vi "Reset Quadrature.vi"(6 "error in":errorcluster, 8 "Reverse?":bool=TRUE, 9 "Forward Position":i32, 10 "Module Number":enum16{"1", "2", "3", "4"}(ring), 11 "CAN Talon SRX Ref":T1={"DeviceStatus"={"status"=FALSE, "code"=0, "source"=""}, "Type"=enum."PWM", "PWM"={"PWM Channel"=enum."PWM 1", "DeadBand"={"Name"="", "maxPositivePwm"=0, "minPositivePwm"=0, "centerPwm"=0, "maxNegativePwm"=0, "minNegativePwm"=0, "angularRange"=0}}, "CAN"={"Device Number"=0, "SetOutput VI Ref"=variant(enum8{"Percent VBus", "Current", "Speed", "Position", "Voltage"} enum."Percent VBus"), "GetOutput VI Ref"=variant(refnum<k1> refnum), "Enable VI Ref"=variant(dbl 12.0), "Disable VI Ref"=variant(enum8{"Percent VBus", "Speed", "Position", "Slave", "Unchanged / Invalid", "Voltage Compensation", "Current", "Motion Profile"} enum."Percent VBus"), "Data"=variant}, "Invert"=FALSE, "DIO PWM"={"PWM \"Enable\" Channel"=enum."Invalid", "DIOChannel"=enum."Invalid", "PWM Rate"=0.0}}) -> (0 "error out":errorcluster, 2 "Motor Output":dbl)   [LabVIEW 2017, in "Huskie Swerve.lvlib"]
uses:
  Huskie Swerve.lvlib
  <vilib>/Rock Robotics/WPI/MotorControl/WPI_MotorControlDeviceRef.ctl
  <vilib>/Rock Robotics/WPI/MotorControl/WPI_MotorControlType.ctl
  <vilib>/Rock Robotics/SystemInterfaces/DIO/FPGA_DIOPWMChannel.ctl
  <vilib>/Rock Robotics/WPI/PWM/WPI_PWMDeadband.ctl
  <vilib>/Rock Robotics/SystemInterfaces/DIO/FPGA_DIOChannel.ctl
  <vilib>/Rock Robotics/WPI/ThirdParty/Phoenix-LabVIEW/Motor Controller/Controls/CTRE_Phoenix_MotorControl_ControlMode.ctl
  <vilib>/Rock Robotics/WPI/ThirdParty/Phoenix-LabVIEW/Motor Controller/Get/CTRE_Phoenix_MotorController_GetPulseWidthAll.vi
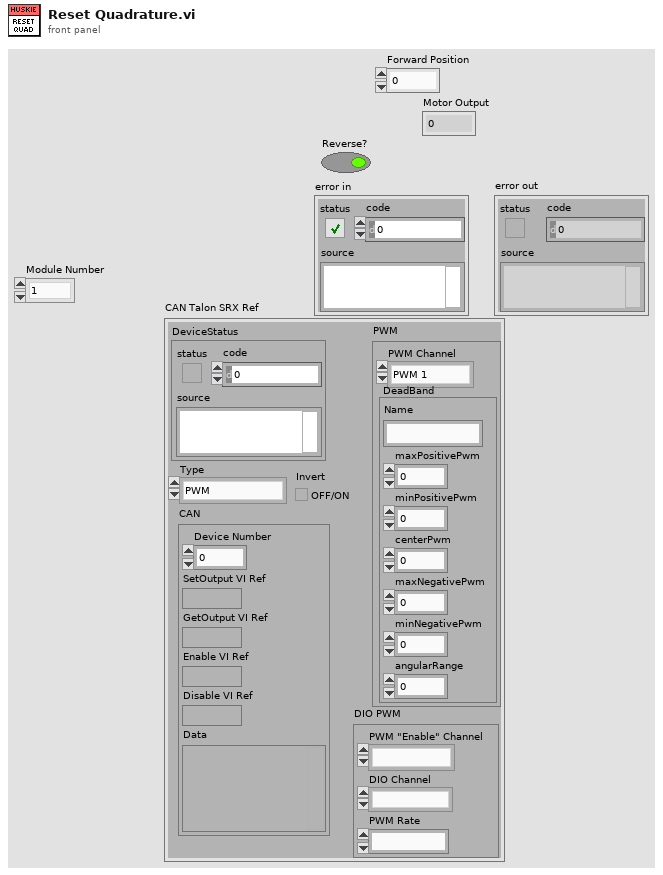
[diagram p1: front panel]
types:
  T1 = typedef "WPI_MotorControlDeviceRef.ctl" = cluster{"DeviceStatus":errorcluster, "Type":T2, "PWM":cluster{"PWM Channel":T3, "DeadBand":T4}, "CAN":cluster{"Device Number":u8, "SetOutput VI Ref":variant, "GetOutput VI Ref":variant, "Enable VI Ref":variant, "Disable VI Ref":variant, "Data":variant}, "Invert":bool, "DIO PWM":cluster{"PWM \"Enable\" Channel":T3, "DIOChannel":T5, "PWM Rate":dbl}}
  T2 = typedef "WPI_MotorControlType.ctl" = enum16{"PWM", "CAN", "DIO PWM"}
  T3 = typedef "FPGA_DIOPWMChannel.ctl" = enum8{"PWM 0", "PWM 1", "PWM 2", "PWM 3", "PWM 4", "PWM 5", "PWM 6", "PWM 7", "PWM 8", "PWM 9", "PWM MXP 0", "PWM MXP 1", "PWM MXP 2", "PWM MXP 3", "PWM MXP 4", "PWM MXP 5", "PWM MXP 6", "PWM MXP 7", "PWM MXP 8", "PWM MXP 9", "Invalid"}
  T4 = typedef "WPI_PWMDeadband.ctl" = cluster{"Name":string, "maxPositivePwm":i32, "minPositivePwm":i32, "centerPwm":i32, "maxNegativePwm":i32, "minNegativePwm":i32, "angularRange":u16}
  T5 = typedef "FPGA_DIOChannel.ctl" = enum8{"DIO 0", "DIO 1", "DIO 2", "DIO 3", "DIO 4", "DIO 5", "DIO 6", "DIO 7", "DIO 8", "DIO 9", "DIO MXP 0", "DIO MXP 1", "DIO MXP 2", "DIO MXP 3", "DIO MXP 4", "DIO MXP 5", "DIO MXP 6", "DIO MXP 7", "DIO MXP 8", "DIO MXP 9", "DIO MXP 10", "DIO MXP 11", "DIO MXP 12", "DIO MXP 13", "DIO MXP 14", "DIO MXP 15", "SPI Port CS1", "SPI Port CS2", "SPI Port CS3", "SPI Port MISO", "SPI Port MOSI", "Invalid"}
  T6 = typedef "CTRE_Phoenix_MotorControl_ControlMode.ctl" = u16
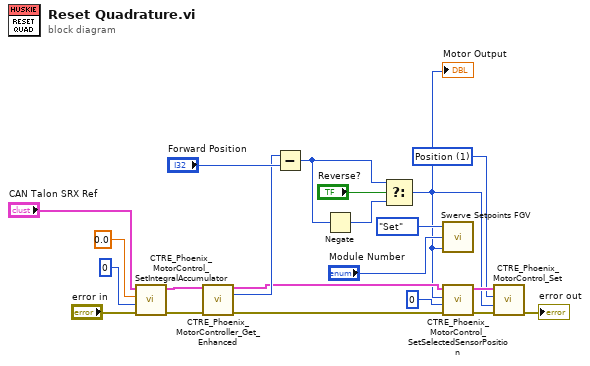
[diagram p0: block diagram]
diagram:
  w3 = T6 1 items=["PercentOutput"=0, "Position"=1, "Velocity"=2, "Current"=3, "Follower"=5, "MotionProfile"=6, "MotionMagic"=7, "MotionMagicArc"=8, "MotionProfileArc"=10, "Disabled"=15] ("Control Mode")
  n1 = call "CTRE_Phoenix_MotorControl_SetIntegralAccumulator.vi"("error in (no error)"="error in", "pidLoopIdx"=u32 0, "Integral Accumulator Value"=0.0, "PhoenixMotorControlDevRef"="CAN Talon SRX Ref") -> ("error out"=w9:errorcluster, "PhoenixMotorControlDevRef"=w10:T1)  [unwired: 6 in]
  n2 = call-poly <vilib>:"CTRE_Phoenix_MotorController_Get_Enhanced.vi"("PhoenixMotorControlDevRef"=w10, "error in"=w9) -> ("PhoenixMotorControlDevRef"=w7:T1, "Pulse Width Position"=w11:i32, "error out"=w6:errorcluster)  [unwired: 8 in, 3 out]
  n3 = Subtract(x=w11, y="Forward Position") -> (x-y=w18:i32)
  n4 = Negate(x=w18) -> (-x=w21:i32)
  n5 = Select(t=w18, s="Reverse?", f=w21) -> (s? t:f=w4:i32)
  "Motor Output" <- w4
  n6 = call "Swerve Setpoints FGV.vi"("New Setpoint"=w4, "Swerve Number"="Module Number", "Action"=enum16{"Set", "Get"}."Set") -> ()  [unwired: 1 out]
  n7 = call "CTRE_Phoenix_MotorControl_SetSelectedSensorPosition.vi"("error in (no error)"=w6, "pidLoopIdx"=u32 0, "New Sensor Position"=w4, "PhoenixMotorControlDevRef"=w7) -> ("error out"=w2:errorcluster, "PhoenixMotorControlDevRef"=w5:T1)  [unwired: 6 in]
  n8 = call "CTRE_Phoenix_MotorControl_Set.vi"("error in (no error)"=w2, "Output"=w4, "Control Mode"=w3, "PhoenixMotorControlDevRef"=w5) -> ("error out"=→"error out":errorcluster)  [unwired: 6 in, 1 out]
